vi "Parse ERD Write Expected Data (Rev 2 API).vi"(0 "ERD Write Data In":T1 {"ERD Number" format="%.0x"}, 5 "Request ID":string, 11 "Error In":errorcluster) -> (8 "Expected Data":string, 15 "Error Out":errorcluster)   [LabVIEW 2019, in "GEA2_Toolkit.lvlib"]
uses:
  library/GEA2_Toolkit.lvlib
  type defs/ERD Write Data In.ctl
  type defs/Data Type.ctl
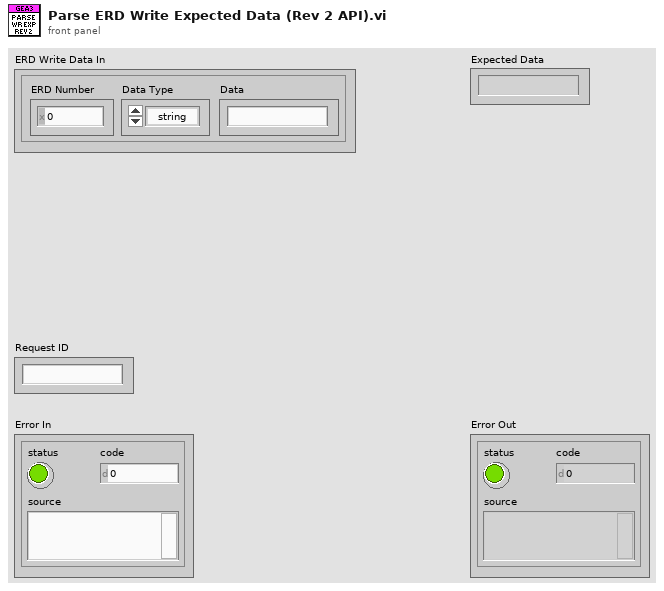
[diagram p1: front panel]
types:
  T1 = typedef "GEA2_Toolkit.lvlib/ERD Write Data In.ctl" = cluster{"ERD Number":u16, "Data Type":T2, "Data":string}
  T2 = typedef "GEA2_Toolkit.lvlib/Data Type.ctl" = enum16{"string", "boolean", "uint8_t", "uint16_t", "uint32_t", "uint64_t", "int8_t", "int16_t", "int32_t", "int64_t"}
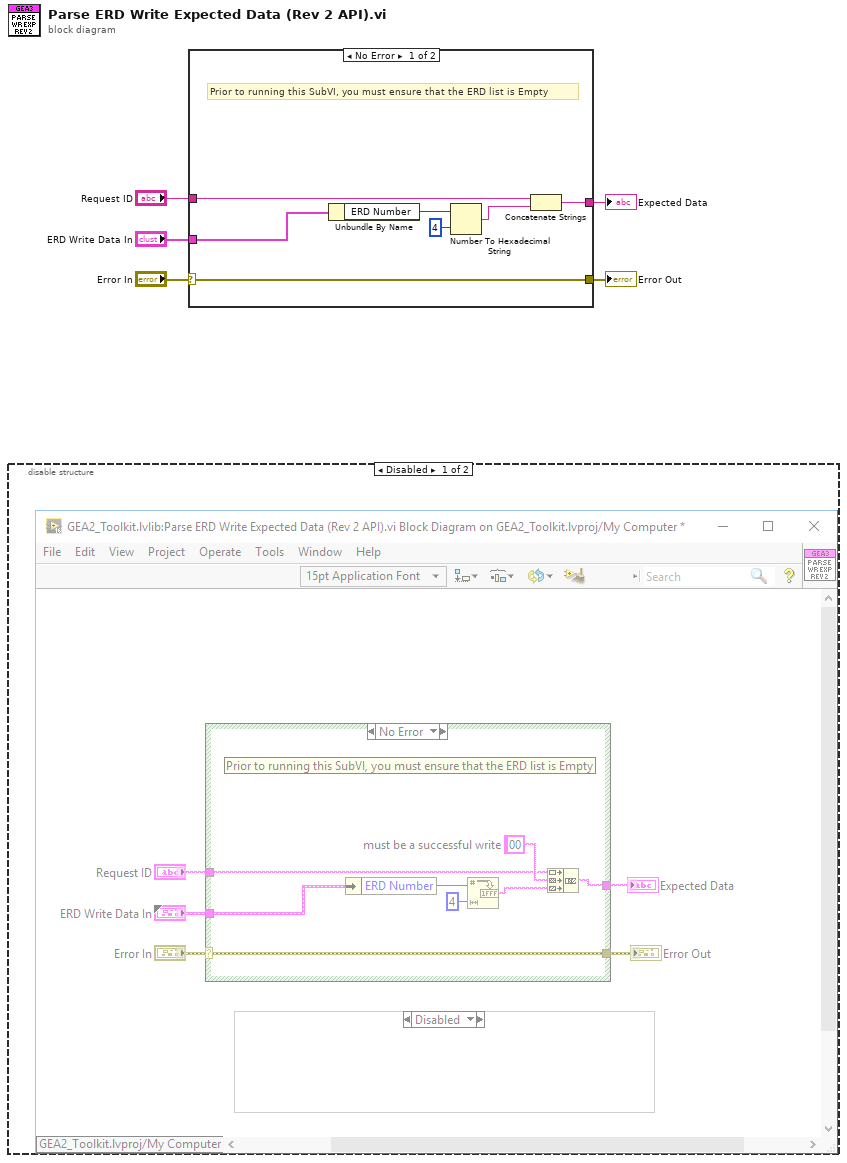
[diagram p0: block diagram]
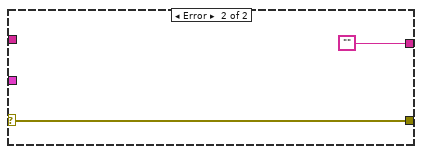
[diagram p3: hidden frame]
diagram:
  n1 = disable-structure shown="Disabled" {
    frame Disabled {
    }
    frame Enabled {
    }
  }
  n2 = case shown="No Error" "Error In" {
    selector: "Error In" -> [w10 w14]
    tunnel: [w11 ""] -> w5
    tunnel: "ERD Write Data In" -> [w6 _]
    tunnel: [w10 w14] -> w3
    tunnel: "Request ID" -> [w7 _]
    frame No Error {
      # "Prior to running this SubVI, you must ensure that the ERD list is Empty"
      n3 = Unbundle By Name(w6) -> ("ERD Number"=w9:u16)
      n4 = Number To Hexadecimal String(1:i16 4 ("width (-)"), 2:w9) -> (0:w12:string)
      n5 = Concatenate Strings(w7, w12) -> (w11:string)
    }
    frame Error {
    }
  }
  "Expected Data" <- w5
  "Error Out" <- w3
